vi "Create Send Thread.vi"(7 "SendQueue":refnum<queue>, 10 "StopNotifier":refnum<notifier>, 11 "Send Data":T1={"Handle"=0, "Frames"=0, "Spare"=0, "Times"=0, "ID+"=FALSE, "Data+"=FALSE, "Type"=enum."CANFD", "Data"=variant}) -> ()   [LabVIEW 2018, in "CAN FD.lvlib"]
uses:
  CAN FD.lvlib
  Typedef/Send Data.ctl
  Send Thread.vi
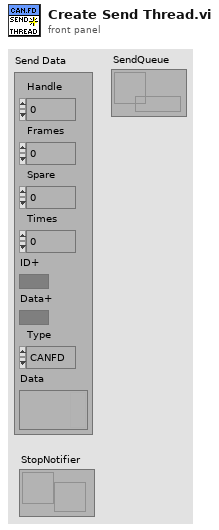
[diagram p1: front panel]
types:
  T1 = typedef "CAN FD.lvlib/Send Data.ctl" = cluster{"Handle":u64, "Frames":u32, "Spare":u32, "Times":i32, "ID+":bool, "Data+":bool, "Type":enum16{"CAN", "CANFD"}, "Data":variant}
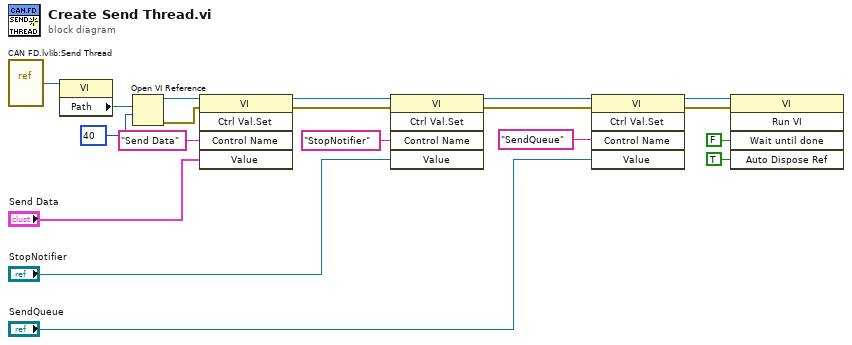
[diagram p0: block diagram]
diagram:
  n1 = vi-ref "CAN FD.lvlib:Send Thread.vi"() -> (w19:refnum<vi>)
  n2 = property class="VI"(reference=w19) -> ("Path"=w18:path)  [unwired: 1 in, 2 out]
  n3 = Open VI Reference(vi path=w18, options=40 ("选项")) -> (vi reference=w16:refnum<vi>, error out=w14:errorcluster)  [unwired: 4 in]
  n4 = invoke class="VI" method="Ctrl Val.Set"(reference=w16, error in=w14, "Control Name"="Send Data" ("控件名"), "Value"="Send Data") -> (reference out=w10:refnum<vi>, error out=w9:errorcluster)  [unwired: 1 in, 3 out]
  n5 = invoke class="VI" method="Ctrl Val.Set"(reference=w10, error in=w9, "Control Name"="StopNotifier" ("控件名"), "Value"="StopNotifier") -> (reference out=w6:refnum<vi>, error out=w5:errorcluster)  [unwired: 1 in, 3 out]
  n6 = invoke class="VI" method="Ctrl Val.Set"(reference=w6, error in=w5, "Control Name"="SendQueue" ("控件名"), "Value"="SendQueue") -> (reference out=w4:refnum<vi>, error out=w3:errorcluster)  [unwired: 1 in, 3 out]
  n7 = invoke class="VI" method="Run VI"(reference=w4, error in=w3, "Wait until done"=FALSE ("结束前等待"), "Auto Dispose Ref"=TRUE ("自动销毁引用")) -> ()  [unwired: 1 in, 5 out]
